vi "-8341 Invalid Lexical Index--error.vi"(8 "error in":errorcluster, 11 "Lexical Index":string) -> (0 "error out":errorcluster)   [LabVIEW 2019, in "Open Xml.lvlib"]
uses:
  Open Xml.lvlib
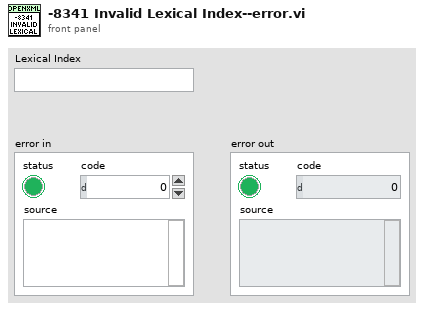
[diagram p1: front panel]
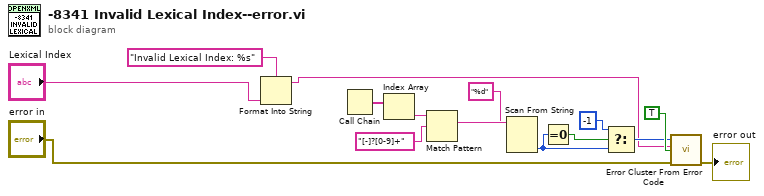
[diagram p0: block diagram]
diagram:
  n1 = Format Into String(format string="Invalid Lexical Index: %s" ("source"), "Lexical Index") -> (resulting string=w10:string)  [unwired: 2 in, 1 out]
  n2 = Call Chain() -> (call chain=w12:string[])
  n3 = Index Array(array=w12) -> (element=w3:string)  [unwired: 1 in]
  n4 = Match Pattern(string=w3, regular expression="[-]?[0-9]+") -> (match substring=w2:string)  [unwired: 1 in, 3 out]
  n5 = Scan From String(format string="%d", input string=w2) -> (output 1=w6:i32)  [unwired: 3 in, 3 out]
  n6 = Equal To 0?(x=w6) -> (x = 0?=w5:bool)
  n7 = Select(t=-1, s=w5, f=w6) -> (s? t:f=w11:i32)
  n8 = call <vilib>:"Error Cluster From Error Code.vi"("show call chain? (False)"=TRUE, "error in (no error)"="error in", "error message (\"\")"=w10, "error code (0)"=w11) -> ("error out"=→"error out":errorcluster)  [unwired: 5 in]
